vi "writeAPDSerial.vi"() -> ()   [LabVIEW 2020]
uses:
  <vilib>/Utility/config.llb/Write Key (String).vi
  <vilib>/Utility/config.llb/NI_LVConfig.lvlib
panel:
  in  "Error In":errorcluster
  out "error out":errorcluster
  in  "APD Serial":T1={"Ch1APDSerial#"="M00562768", "Ch2APDSerial#"="M00549707", "Ch3APDSerial#"="M00549708"}
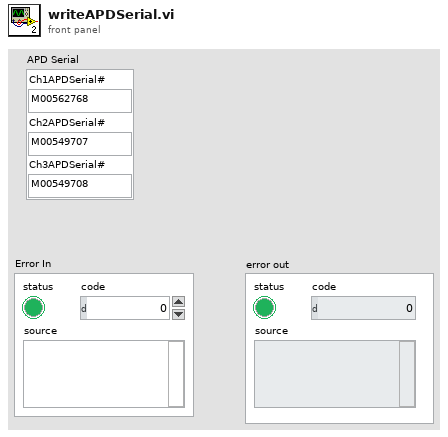
[diagram p1: front panel]
types:
  T1 = cluster{"Ch1APDSerial#":string, "Ch2APDSerial#":string, "Ch3APDSerial#":string}
  T2 = typedef "NI_LVConfig.lvlib/Config Data RefNum.ctl" = refnum<k1>
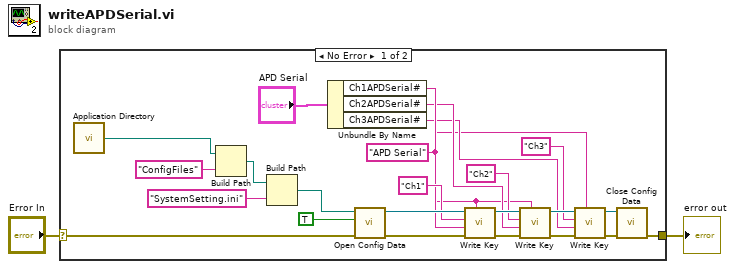
[diagram p0: block diagram]
diagram:
  n1 = case shown="No Error" "Error In" {
    selector: "Error In" -> [w21 w27]
    tunnel: [w8 w27] -> w2
    frame No Error {
      w3 = "APD Serial" ("section")
      n2 = call <vilib>:"Application Directory.vi"() -> ("Application Directory"=w26:path)
      n3 = Build Path(base path=w26, name or relative path="ConfigFiles") -> (appended path=w24:path)
      n4 = Build Path(base path=w24, name or relative path="SystemSetting.ini") -> (appended path=w11:path)
      n5 = Unbundle By Name("APD Serial") -> ("Ch1APDSerial#"=w6:string, "Ch2APDSerial#"=w5:string, "Ch3APDSerial#"=w4:string)
      n6 = call <vilib>:"Open Config Data.vi"("error in (no error)"=w21, "create file if necessary (T)"=TRUE, "configuration file path"=w11) -> ("error out"=w19:errorcluster, "refnum"=w20:T2)  [unwired: 6 in, 1 out]
      n7 = call-poly <vilib>:"Write Key.vi"("section"=w3, "error in (no error)"=w19, "value"=w6, "key"="Ch1", "refnum"=w20) -> ("error out"=w17:errorcluster, "refnum out"=w18:T2)  [unwired: 4 in, 1 out]
      n8 = call-poly <vilib>:"Write Key.vi"("section"=w3, "error in (no error)"=w17, "value"=w5, "key"="Ch2", "refnum"=w18) -> ("error out"=w15:errorcluster, "refnum out"=w16:T2)  [unwired: 4 in, 1 out]
      n9 = call-poly <vilib>:"Write Key.vi"("section"=w3, "error in (no error)"=w15, "value"=w4, "key"="Ch3", "refnum"=w16) -> ("error out"=w9:errorcluster, "refnum out"=w10:T2)  [unwired: 4 in, 1 out]
      n10 = call <vilib>:"Close Config Data.vi"("error in (no error)"=w9, "refnum"=w10) -> ("error out"=w8:errorcluster)  [unwired: 8 in, 1 out]
    }
    frame Error {
    }
  }
  "error out" <- w2
